vi "Get Alarm  Error Status.vi"() -> (1 "AlarmStatus":string, 2 "ErrorStatus":string)   [LabVIEW 2017]
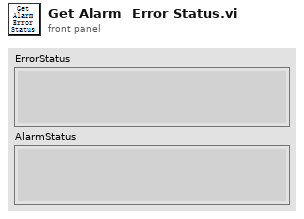
[diagram p1: front panel]
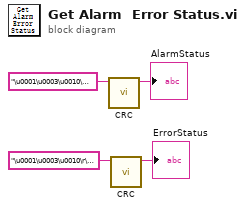
[diagram p0: block diagram]
diagram:
  n1 = call "CRC.vi"("字符串"="\u0001\u0003\u0010\u0005\u0000\u0001") -> ("连接的字符串"=→"AlarmStatus":string)  [unwired: 9 in, 1 out]
  n2 = call "CRC.vi"("字符串"="\u0001\u0003\u0010\r\u0000\u0001") -> ("连接的字符串"=→"ErrorStatus":string)  [unwired: 9 in, 1 out]
